vi "Check if Valid.vi"(5 "produce error if invalid (F)":bool, 7 "chain levels to remove (2)":i32=2 min=2, 8 "error in (no error)":errorcluster, 11 "motor communication in":refnum<class "NI_Robotics_Motor Communication.lvclass">) -> (0 "error out":errorcluster, 2 "valid?":bool, 3 "motor communication out":refnum<class "NI_Robotics_Motor Communication.lvclass">)   [LabVIEW 2017, in "NI_Robotics_Motor Communication.lvclass"]
uses:
  <vilib>/robotics/Actuation/Motor Communication/NI_Robotics_Motor Communication.lvclass
  <vilib>/robotics/Utilities/NI_Robotics Utilities.lvlib
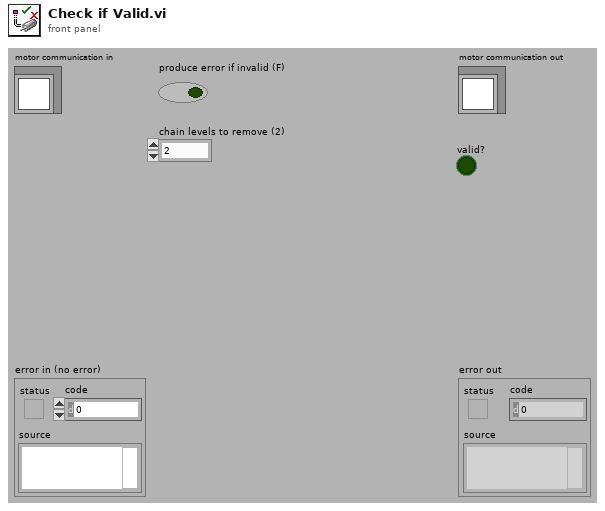
[diagram p1: front panel]
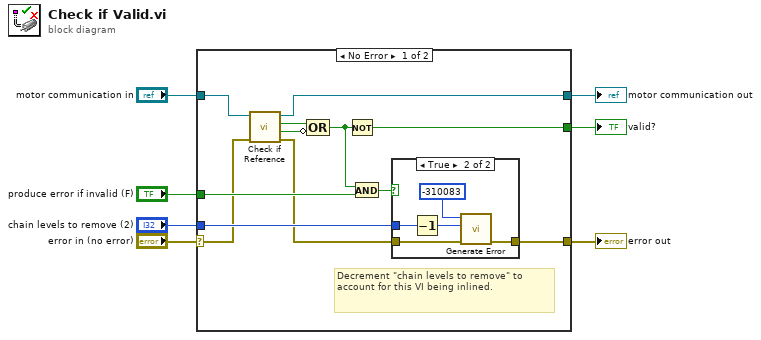
[diagram p0: block diagram]
diagram:
  n1 = case shown="No Error" "error in (no error)" {
    selector: "error in (no error)" -> [w11 w27]
    tunnel: [w17 w27] -> w6
    tunnel: [w8 w26] -> w4
    tunnel: "motor communication in" -> [w9 w26]
    tunnel: [w19 _] -> w3
    tunnel: "produce error if invalid (F)" -> [w18 _]
    tunnel: "chain levels to remove (2)" -> [w15 _]
    frame No Error {
      # "Decrement \"chain levels to remove\" to account for this VI being inlined."
      n2 = call-dynamic "Check if Reference.vi"("error in (no error)"=w11, "motor communication in"=w9) -> ("error out"=w10:errorcluster, "initialized?"=w13:bool, "invalid refs?"=w14:bool, "motor communication out"=w8:refnum<class "NI_Robotics_Motor Communication.lvclass">)  [unwired: 6 in]
      n3 = Compound Arithmetic op=OR(w14, invert w13) -> (w12:bool)
      n4 = Not(x=w12) -> (.not. x?=w19:bool)
      n5 = And(x=w12, y=w18) -> (x .and. y?=w16:bool)
      n6 = case shown="True" w16 {
        tunnel: w10 -> [w20 w25]
        tunnel: [w20 w24] -> w17
        tunnel: w15 -> [_ w22]
        frame False {
        }
        frame True {
          n7 = Decrement(x=w22) -> (x-1=w21:i32)
          n8 = call <vilib>:"Generate Error.vi"("error in (no error)"=w25, "chain levels to remove (1)"=w21, "code"=-310083) -> ("error out"=w24:errorcluster)  [unwired: 8 in]
        }
      }
    }
    frame Error {
    }
  }
  "error out" <- w6
  "motor communication out" <- w4
  "valid?" <- w3
